vi "Drive Code or Whatever Crap.vi"(0 "Right Actual":dbl, 1 "TankDriveEnum":T1, 2 "HalfDrive":bool, 3 "StraightDrive":bool, 5 "LeftActual":dbl, 7 "MotorName":string="TankDrive", 9 "RightDesired":dbl, 11 "LeftDesired":dbl, 12 "error in (no error)":errorcluster) -> (4 "RightOut":dbl, 6 "LeftOut":dbl, 14 "error out":errorcluster)   [LabVIEW 2013]
doc: "Straight drive True locks both motor desired values to the left joystick.\nHalf drive True divides desired values by 2 to allow more fine controls. This does not half the accel rate."
uses:
  TankDriveEnum.ctl
  <vilib>/Rock Robotics/WPI/RobotDrive/WPI_RobotDriveGetSetRefNum.vi
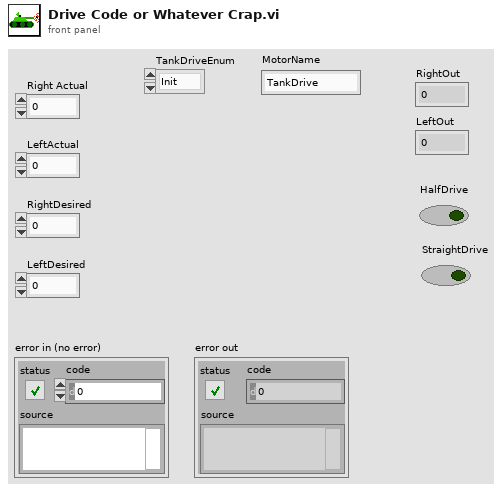
[diagram p1: front panel]
types:
  T1 = typedef "TankDriveEnum.ctl" = enum16{"Init", "SetValue", "Disable"}
  T2 = typedef "WPI_RobotDriveDevRef.ctl" = cluster{"DevStatus":errorcluster, "Motors[]":T3[], "Square Inputs":bool, "Max Output":dbl, "Isochronous":bool}
  T3 = typedef "WPI_MotorControlDeviceRef.ctl" = cluster{"DeviceStatus":errorcluster, "Type":enum16{"PWM", "CAN"}, "PWM":cluster{"Digital Module":T4, "PWM Channel":T5, "DeadBand":T6}, "CAN":cluster{"Device Number":u8, "Control Mode":T7, "Semaphore":T8, "Max Vout":dbl}, "Invert":bool, "TransformRef":T9, "InvTransformRef":T9}
  T4 = typedef "FPGA_TypedefDigitalModule.ctl" = enum16{"Digital Module 1", "Digital Module 2"}
  T5 = typedef "FPGA_DIOPWMChannel.ctl" = enum8{"PWM 1", "PWM 2", "PWM 3", "PWM 4", "PWM 5", "PWM 6", "PWM 7", "PWM 8", "PWM 9", "PWM 10", "Invalid"}
  T6 = typedef "WPI_PWMDeadband.ctl" = cluster{"Name":string, "maxPositivePwm":i32, "minPositivePwm":i32, "centerPwm":i32, "maxNegativePwm":i32, "minNegativePwm":i32, "angularRange":u16}
  T7 = typedef "WPI_CANJaguar_ControlMode.ctl" = enum8{"Percent VBus", "Current", "Speed", "Position", "Voltage"}
  T8 = typedef "Semaphore RefNum" = refnum<k1>
  T9 = typedef "WPI_PWMTransform_ConPane.ctl" = refnum<vi>
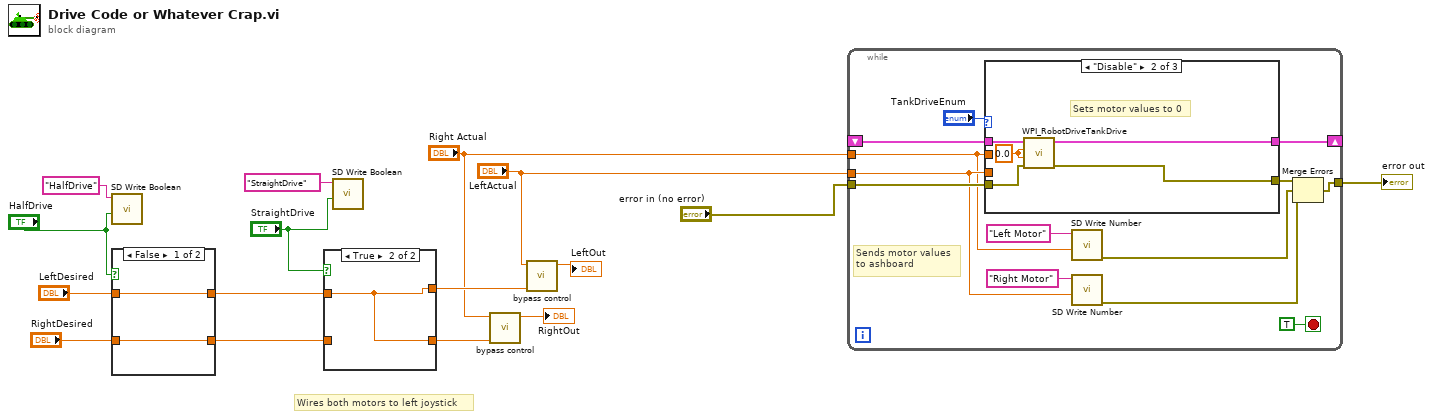
[diagram p0: block diagram]
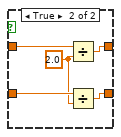
[diagram p3: hidden frame]
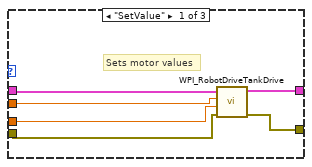
[diagram p4: hidden frame]
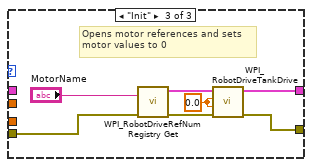
[diagram p5: hidden frame]
diagram:
  # "Wires both motors to left joystick"
  n1 = call <vilib>:"SD Write Boolean.vi"("Boolean"="HalfDrive", "Name"="HalfDrive") -> ()  [unwired: 8 in, 2 out]
  n2 = case shown="False" "HalfDrive" {
    tunnel: "LeftDesired" -> [w18 w23]
    tunnel: "RightDesired" -> [w17 w22]
    tunnel: [w18 w20] -> w6
    tunnel: [w17 w19] -> w8
    frame False {
    }
    frame True {
      w21 = 2.0
      n3 = Divide(x=w23, y=w21) -> (x/y=w20:dbl)
      n4 = Divide(x=w22, y=w21) -> (x/y=w19:dbl)
    }
  }
  n5 = case shown="True" "StraightDrive" {
    tunnel: [w25 w26] -> w5
    tunnel: w8 -> [w25 _]
    tunnel: [w24 w26] -> w7
    tunnel: w6 -> [w24 w26]
    frame False {
    }
    frame True {
    }
  }
  n6 = call <vilib>:"SD Write Boolean.vi"("Boolean"="StraightDrive", "Name"="StraightDrive") -> ()  [unwired: 8 in, 2 out]
  n7 = call "bypass control.vi"("Joystick"=w5, "MotorInput"="Right Actual") -> ("SetMotor"=→"RightOut":dbl)  [unwired: 9 in]
  n8 = call "bypass control.vi"("Joystick"=w7, "MotorInput"="LeftActual") -> ("SetMotor"=→"LeftOut":dbl)  [unwired: 9 in]
  n9 = while {
    shift-right: [w39] -> _
    shift-left: _ -> [w37]
    tunnel: [w30] -> w16
    tunnel: "error in (no error)" -> [w35]
    tunnel: "LeftActual" -> [w28]
    tunnel: "Right Actual" -> [w27]
    stop <- TRUE stop-if-true
    # "Sends motor values\nto ashboard"
    n10 = case shown="\"Disable\"" "TankDriveEnum" {
      tunnel: [w44 w49 w56] -> w39
      tunnel: w37 -> [w45 w50 _]
      tunnel: w35 -> [w43 w47 w54]
      tunnel: [w42 w46 w52] -> w31
      tunnel: w27 -> [w41 _ _]
      tunnel: w28 -> [w40 _ _]
      frame "SetValue" {
        # "Sets motor values"
        n11 = call <vilib>:"WPI_RobotDriveTankDrive.vi"("error in (no error)"=w43, "Right axis value"=w40, "Left axis value"=w41, "RobotDriveDevRef"=w45) -> ("error out"=w42:errorcluster, "RobotDriveDevRef"=w44:T2)  [unwired: 5 in, 1 out]
      }
      frame "Disable" {
        w48 = 0.0
        # "Sets motor values to 0"
        n12 = call <vilib>:"WPI_RobotDriveTankDrive.vi"("error in (no error)"=w47, "Right axis value"=w48, "Left axis value"=w48, "RobotDriveDevRef"=w50) -> ("error out"=w46:errorcluster, "RobotDriveDevRef"=w49:T2)  [unwired: 5 in, 1 out]
      }
      frame "Init" {
        w55 = 0.0
        # "Opens motor references and sets\nmotor values to 0"
        n13 = call <vilib>:"WPI_RobotDriveRefNum Registry Get.vi"("error in (no error)"=w54, "refnum name"="MotorName") -> ("error out"=w53:errorcluster, "RobotDriveDevRef"=w57:T2)  [unwired: 8 in]
        n14 = call <vilib>:"WPI_RobotDriveTankDrive.vi"("error in (no error)"=w53, "Right axis value"=w55, "Left axis value"=w55, "RobotDriveDevRef"=w57) -> ("error out"=w52:errorcluster, "RobotDriveDevRef"=w56:T2)  [unwired: 5 in, 1 out]
      }
    }
    n15 = call <vilib>:"SD Write Number.vi"("Numeric"=w27, "Name"="Left Motor") -> ("error out"=w32:errorcluster)  [unwired: 8 in, 1 out]
    n16 = call <vilib>:"SD Write Number.vi"("Numeric"=w28, "Name"="Right Motor") -> ("error out"=w29:errorcluster)  [unwired: 8 in, 1 out]
    n17 = Merge Errors(w31, w32, w29) -> (w30:errorcluster)
  }
  "error out" <- w16
